vi "TestServer.vi"() -> ()   [LabVIEW 2016]
uses:
  AalborgServerModes.ctl
panel:
  in  "Gas Release System":string="GRC-A"
  out "Output":cluster{"Start":dbl, "ServerMessages":string}[](array[cluster])
  in  "Multiplier":dbl=0.3
  in  "End":dbl=350.0
  in  "Start":dbl=1.0
  in  "Pause(s)":u32=5
  out "ServerMessages":string="\t\t\t\t\t\t\t\t\t\n"
  out "Q[Total]:Dem(l/min)":dbl min=0.0 max=360.0 step=1.0 format="%.2f"
  in  "Temperature channel":string="MFCcal:Temp:(C)"
  in  "Pressure channel":string="CSU:Pressure:mBar"
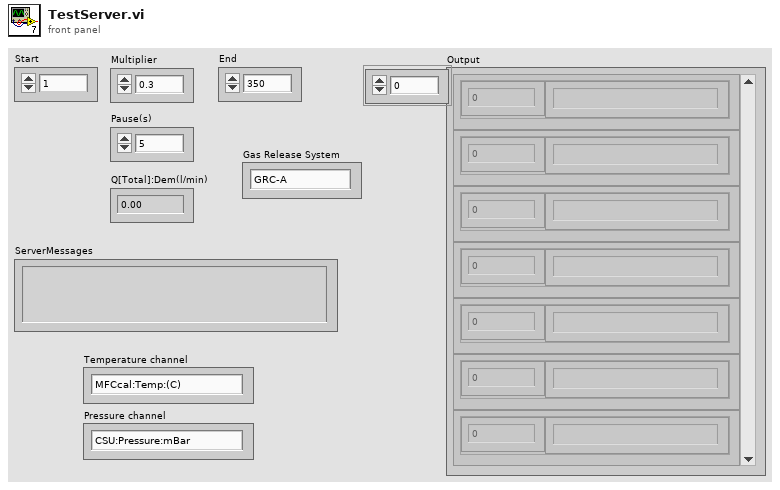
[diagram p1: front panel]
types:
  T1 = typedef "AalborgServerModes.ctl" = enum16{"Set Flows", "Check Flows Are Achievable", "Close All MFCs"}
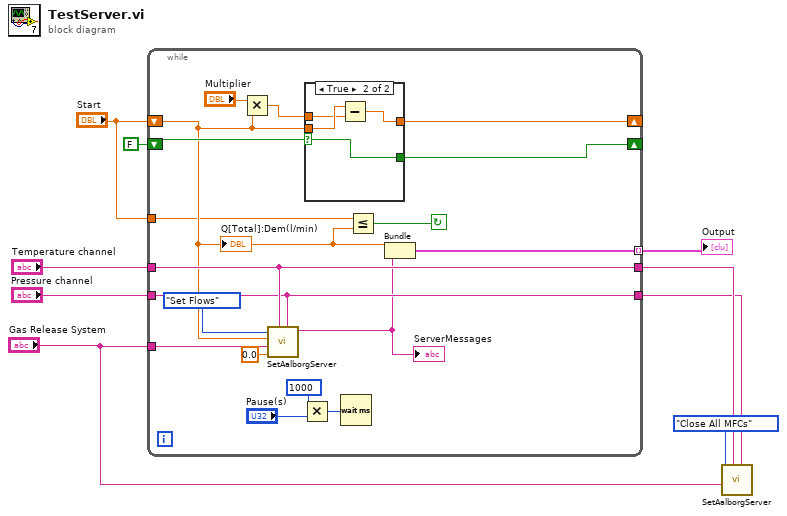
[diagram p0: block diagram]
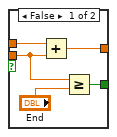
[diagram p2: hidden frame]
diagram:
  n1 = while {
    shift-right: [w25] -> _
    shift-left: "Start" -> [w11]
    tunnel: [w19] -> w9 mode=indexing
    tunnel: "Temperature channel" -> [w18]
    tunnel: [w18] -> w7
    tunnel: "Pressure channel" -> [w17]
    tunnel: [w17] -> w5
    tunnel: "Gas Release System" -> [w16]
    shift-right: [w13] -> _
    shift-left: FALSE -> [w14]
    tunnel: "Start" -> [w10]
    stop <- w12 continue-if-true
    n2 = Multiply(x="Multiplier", y=w11) -> (x*y=w26:dbl)
    n3 = call "SetAalborgServer.vi"("Pressure channel"=w17, "Temperature channel"=w18, "C:Dem(%)"=0.0, "Gas Release System"=w16, "Q[Total]:Dem(l/min)"=w11, "Mode"=AalborgServerModes."Set Flows") -> ("ErrorString"=w15:string)  [unwired: 4 in, 1 out]
    "ServerMessages" <- w15
    n4 = Multiply(x=u32 1000, y="Pause(s)") -> (x*y=w21:u32)
    n5 = case shown="True" w14 {
      selector: w14 -> [_ w36]
      tunnel: w26 -> [w32 w33]
      tunnel: [w31 w35] -> w25
      tunnel: w11 -> [w29 w34]
      tunnel: [w28 w36] -> w13
      frame False {
        n6 = Add(x=w32, y=w29) -> (x+y=w31:dbl)
        n7 = Greater Or Equal?(x=w29, y="End") -> (x >= y?=w28:bool)
      }
      frame True {
        n8 = Subtract(x=w34, y=w33) -> (x-y=w35:dbl)
      }
    }
    n9 = Wait (ms)(milliseconds to wait=w21) -> ()  [unwired: 1 out]
    n10 = Less Or Equal?(x=w10, y=w11) -> (x <= y?=w12:bool)
    n11 = Bundle("Start"=w11, "ErrorString"=w15) -> (w19:cluster{"Start":dbl, "ErrorString":string})  [unwired: 1 in]
    "Q[Total]:Dem(l/min)" <- w11
  }
  "Output" <- w9
  n12 = call "SetAalborgServer.vi"("Pressure channel"=w5, "Temperature channel"=w7, "Gas Release System"="Gas Release System", "Mode"=AalborgServerModes."Close All MFCs") -> ()  [unwired: 6 in, 2 out]
